vi "Overwrite ID.vi"(8 "error in (no error)":errorcluster, 10 "Numeric":i32, 11 "String":string) -> (0 "error out":errorcluster, 3 "<JSON>":string)   [LabVIEW 2023, in "Communicator.lvclass"]
doc: "Overwrites the message ID if a custom ID is to be used for messaging to the ICL."
uses:
  Communicator.lvclass
  bc487742-c063-4e24-9239-0c2f1fdaf8c9.vi
  <vilib>/JDP Science/JSONtext/Variant to JSON Text.vi
  <vilib>/JDP Science/JSONtext/Set Item.vi
  <vilib>/JDP Science/JSONtext/LVClass Serializer/JSONtext LVClass Serializer.lvclass
  <vilib>/JDP Science/JSONtext/JSONtext.lvlib
panel:
  # "Connector Pane"
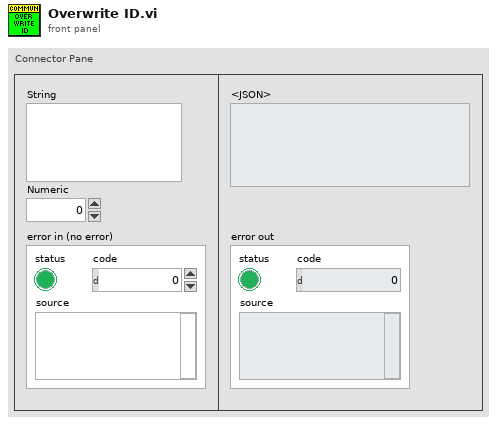
[diagram p1: front panel]
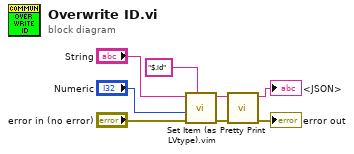
[diagram p0: block diagram]
diagram:
  n1 = call "Set Item (as LVtype).vim"("$Path or Item Name"="$.id", "error in (no error)"="error in (no error)", "Anything"="Numeric", "JSON"="String") -> ("error out"=w7:errorcluster, "<JSON>"=w5:string)  [unwired: 4 in, 1 out]
  n2 = call <vilib>:"Pretty Print.vi"("error in (no error)"=w7, "JSON"=w5) -> ("error out"=→"error out":errorcluster, "<JSON>"=→"<JSON>":string)  [unwired: 7 in, 1 out]
